vi "LocalAppData Get Base Path.vi"(8 "error in (no error)":errorcluster) -> (0 "error out":errorcluster, 3 "Path":path)   [LabVIEW 2020, in "RxnRover.lvlib" / "File IO.lvlib" / "LocalAppData Utilities.lvlib"]
doc: "Uses command prompt based off of the current operating system to retrive the LocalAppData base path\nSupports: Windows 2000 - Windows 11, Linux, Mac OS\n\nCreated 5/20/2025 - Labview 2020\nRxnRover"
uses:
  LocalAppData Utilities.lvlib
  <vilib>/Utility/sysdir.llb/System Directory Type.ctl
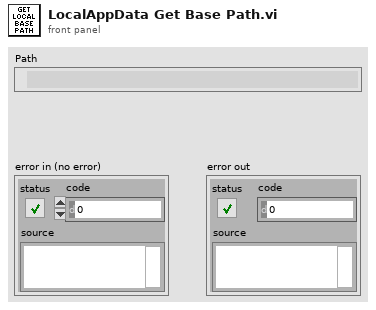
[diagram p1: front panel]
types:
  T1 = typedef "System Directory Type.ctl" = i32
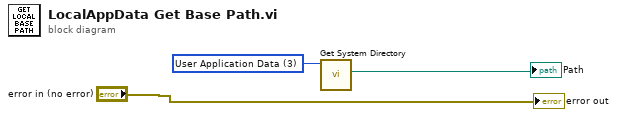
[diagram p0: block diagram]
diagram:
  w1 = T1 3 items=["User Home"=0, "User Desktop"=1, "User Documents"=2, "User Application Data"=3, "User Preferences"=4, "User Temporary"=5, "Public Documents"=6, "Public Application Data"=7, "Public Preferences"=8, "Public Cache"=13, "System Core Libraries"=9, "System Installed Libraries"=10, "Application Files"=11, "Boot Volume Root"=12] ("system directory type")
  n1 = call <vilib>:"Get System Directory.vi"("system directory type"=w1) -> ("system directory"=→"Path":path)  [unwired: 10 in]
  "error out" <- "error in (no error)"
